vi "Search for Unit or Greek Letter.vi"(0 "Text":string, 11 "error in (no error)":errorcluster) -> (4 "Text OUT":string, 8 "Text [ ]":string[](array[string]), 15 "error out":errorcluster)   [LabVIEW 2019]
doc: "Developed by Jean-Marc Simard\nCopyright © 2012, Exaprom Inc.\nAll rights reserved.\nLicense: BSD\n\nWith iTextSharp 4.1.6 (http://itextsharp.sourceforge.net)\nunder Mozilla Public License Version 1.1\n(http://www.mozilla.org/MPL/MPL-1.1.html)"
uses:
  <vilib>/regexp/Match Regular Expression.xnode
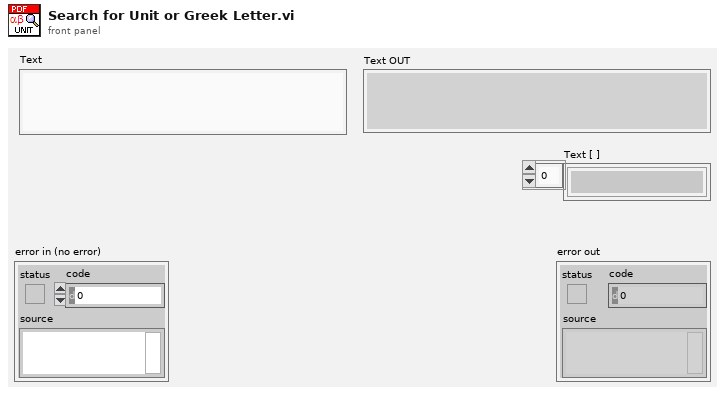
[diagram p1: front panel]
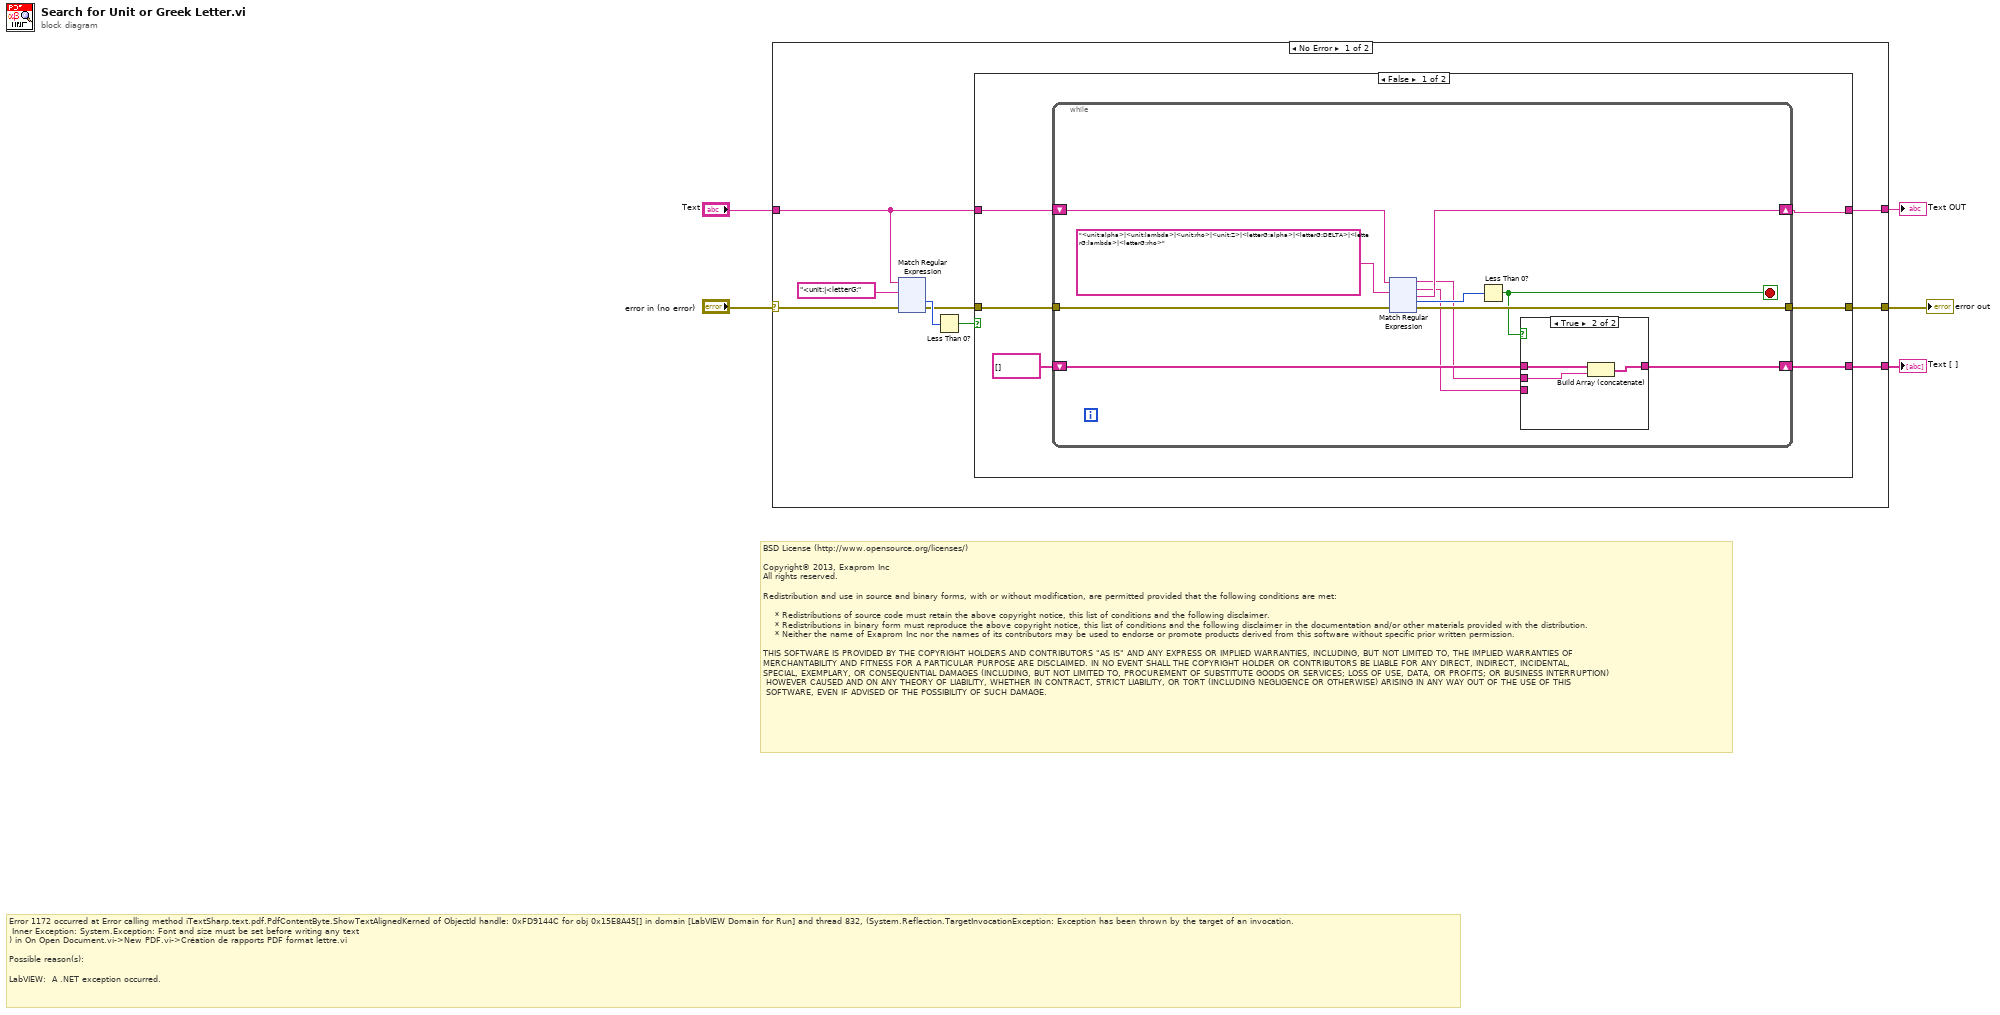
[diagram p0: block diagram]
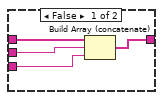
[diagram p2: hidden frame]
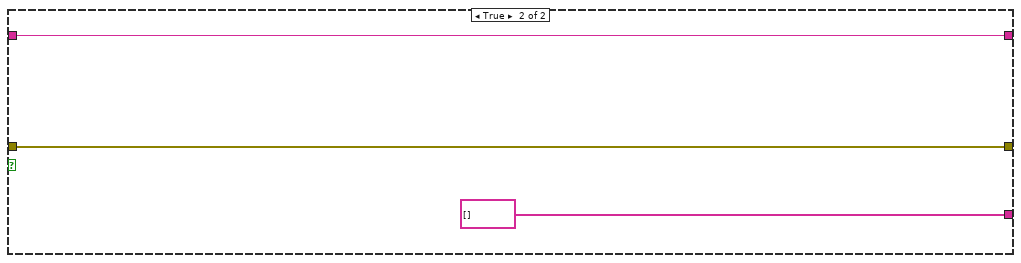
[diagram p3: hidden frame]
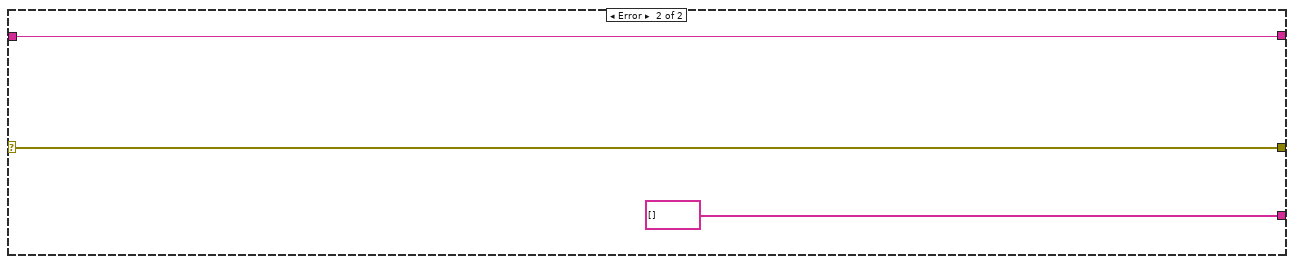
[diagram p4: hidden frame]
diagram:
  # "Error 1172 occurred at Error calling method iTextSharp.text.pdf.PdfContentByte.ShowTextAlignedKerned of ObjectId handle: 0xFD9144C for obj 0x15E8A45[] in domain [LabVIEW Domain for Run] and thread 832, (System.Reflection.TargetInvocationException: Exception has been thrown by the target of an invocation.\n\tInner Exception: System.Exception: Font and size must be set before writing any text\n) in On Open Document.vi->New PDF.vi->Création de rapports PDF format lettre.vi\n\nPossible reason(s):\n\nLabVIEW:  A .NET exception occurred."
  # "BSD License (http://www.opensource.org/licenses/)\n\nCopyright© 2013, Exaprom Inc\nAll rights reserved.\n\nRedistribution and use in source and binary forms, with or without modification, are permitted provided that the following conditions are met:\n\n    * Redistributions of source code must retain the above copyright notice, this list of conditions and the following disclaimer.\n    * Redistributions in binary form must reproduce the above copyright notice, this list of conditions and the following disclaimer in the documentation and/or other materials provided with the distribution.\n    * Neither the name of Exaprom Inc nor the names of its contributors may be used to endorse or promote products derived from this software without specific prior written permission.\n\nTHIS SOFTWARE IS PROVIDED BY THE COPYRIGHT HOLDERS AND CONTRIBUTORS \"AS IS\" AND ANY EXPRESS OR IMPLIED WARRANTIES, INCLUDING, BUT NOT LIMITED TO, THE IMPLIED WARRANTIES OF \nMERCHANTABILITY AND FITNESS FOR A PARTICULAR PURPOSE ARE DISCLAIMED. IN NO EVENT SHALL THE COPYRIGHT HOLDER OR CONTRIBUTORS BE LIABLE FOR ANY DIRECT, INDIRECT, INCIDENTAL,\nSPECIAL, EXEMPLARY, OR CONSEQUENTIAL DAMAGES (INCLUDING, BUT NOT LIMITED TO, PROCUREMENT OF SUBSTITUTE GOODS OR SERVICES; LOSS OF USE, DATA, OR PROFITS; OR BUSINESS INTERRUPTION)\n HOWEVER CAUSED AND ON ANY THEORY OF LIABILITY, WHETHER IN CONTRACT, STRICT LIABILITY, OR TORT (INCLUDING NEGLIGENCE OR OTHERWISE) ARISING IN ANY WAY OUT OF THE USE OF THIS\n SOFTWARE, EVEN IF ADVISED OF THE POSSIBILITY OF SUCH DAMAGE."
  n1 = case shown="No Error" "error in (no error)" {
    selector: "error in (no error)" -> [w13 w272]
    tunnel: [w7 w272] -> w5
    tunnel: "Text" -> [w8 w271]
    tunnel: [w9 w271] -> w2
    tunnel: [w6 string[] []] -> w1
    frame No Error {
      n2 = xnode "Match Regular Expression"("input string"=w8, "regular expression"="<unit:|<letterG:", "error in"=w13) -> ("offset past match"=w12:i32, "error out"=w10:errorcluster)  [unwired: 3 in, 3 out]
      n3 = Less Than 0?(x=w12) -> (x < 0?=w11:bool)
      n4 = case shown="False" w11 {
        tunnel: w10 -> [w19 w154]
        tunnel: [w16 w155] -> w9
        tunnel: w8 -> [w20 w155]
        tunnel: [w18 w154] -> w7
        tunnel: [w15 string[] []] -> w6
        frame False {
          n5 = while {
            shift-right: [w28] -> w16
            shift-left: w20 -> [w30]
            tunnel: w19 -> [w31]
            tunnel: [w26] -> w18
            shift-right: [w23] -> w15
            shift-left: string[] [] -> [w24]
            stop <- w25 stop-if-true
            n6 = xnode "Match Regular Expression"("input string"=w30, "regular expression"="<unit:alpha>|<unit:lambda>|<unit:rho>|<unit:Z>|<letterG:alpha>|<letterG:DELTA>|<letterG:lambda>|<letterG:rho>", "error in"=w31) -> ("before match"=w22:string, "whole match"=w21:string, "after match"=w28:string, "offset past match"=w27:i32, "error out"=w26:errorcluster)  [unwired: 3 in]
            n7 = Less Than 0?(x=w27) -> (x < 0?=w25:bool)
            n8 = case shown="True" w25 {
              tunnel: w24 -> [w35 w38]
              tunnel: [w34 w37] -> w23
              tunnel: w22 -> [w33 w36]
              tunnel: w21 -> [w32 _]
              frame False {
                n9 = Build Array (concatenate)(w35, w33, w32) -> (w34:string[])
              }
              frame True {
                n10 = Build Array (concatenate)(w38, w36) -> (w37:string[])
              }
            }
          }
        }
        frame True {
        }
      }
    }
    frame Error {
    }
  }
  "error out" <- w5
  "Text OUT" <- w2
  "Text [ ]" <- w1
